vi "Serialize - Text.vi"(8 "error in":errorcluster, 11 "ePAS Cell Data in":refnum<class "ePAS Cell Data.lvclass">) -> (0 "error out":errorcluster, 2 "Serialized Text":string, 3 "ePAS Cell Data out":refnum<class "ePAS Cell Data.lvclass">)   [LabVIEW 2014, in "ePAS Library.lvlib" / "ePAS Cell Data.lvclass"]
uses:
  ePAS Cell Data.lvclass
  ePAS Cell Data.lvclass/ePAS Cell Data.ctl
  reusable/PAS/Data/Cell/PAS Cell Data.lvclass
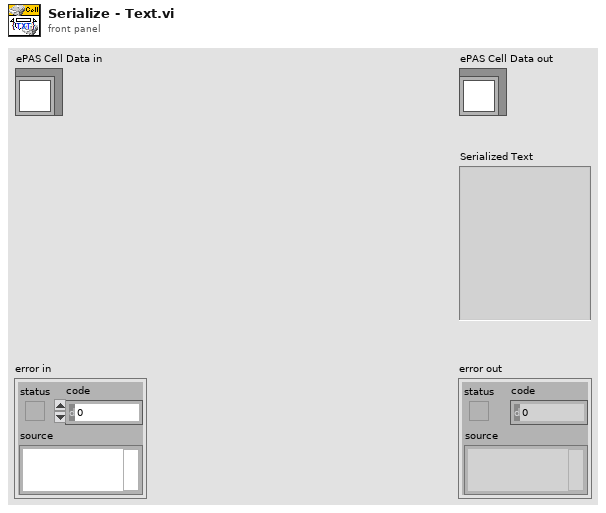
[diagram p1: front panel]
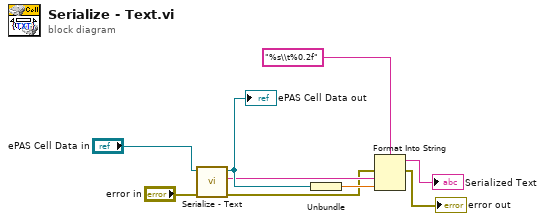
[diagram p0: block diagram]
diagram:
  n1 = call-parent "Serialize - Text.vi"("error in"="error in", "PAS Cell Data in"="ePAS Cell Data in") -> ("error out"=w2:errorcluster, "Serialized Text"=w6:string, "PAS Cell Data out"=w7:refnum<class "ePAS Cell Data.lvclass">)  [unwired: 7 in]
  "ePAS Cell Data out" <- w7
  n2 = Unbundle(w7) -> (w4:dbl)
  n3 = Format Into String(format string="%s\\t%0.2f", error in=w2, w6, w4) -> (resulting string=→"Serialized Text":string, error out=→"error out":errorcluster)  [unwired: 1 in]
